vi "deserialize (Frames-AIM).vi"(11 "data in":string[][](array[string])) -> (3 "frames":map{string, map{string, T1}}[](array[numeric]))   [LabVIEW 2020]
uses:
  _controls/1553_minorFrames.ctl
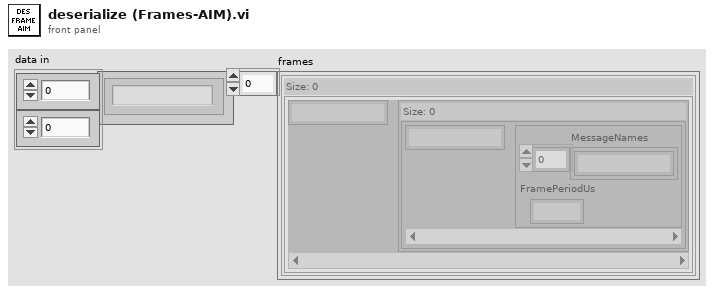
[diagram p1: front panel]
types:
  T1 = typedef "1553_minorFrames.ctl" = cluster{"MessageNames":string[], "FramePeriodUs":i32}
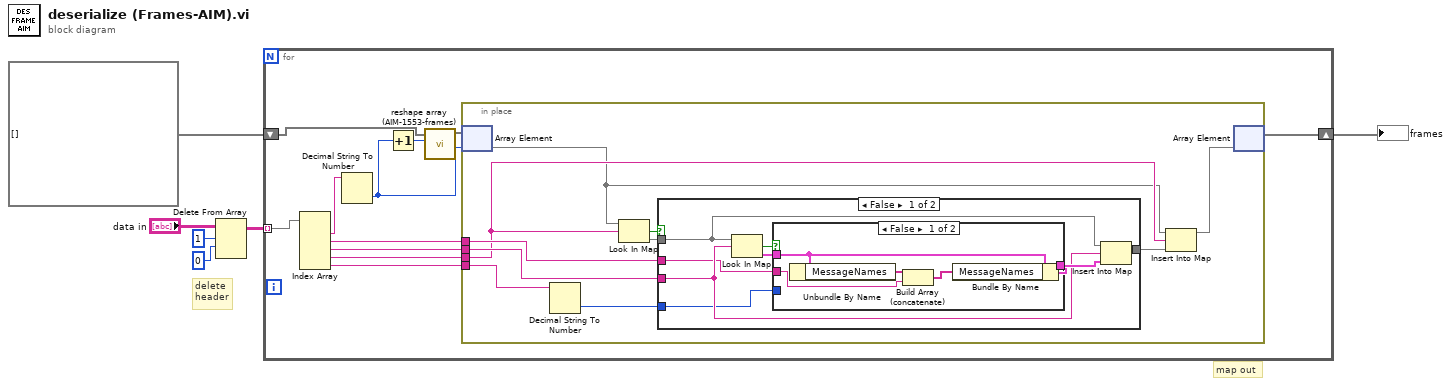
[diagram p0: block diagram]
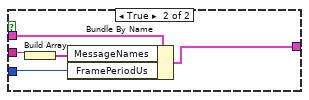
[diagram p2: hidden frame]
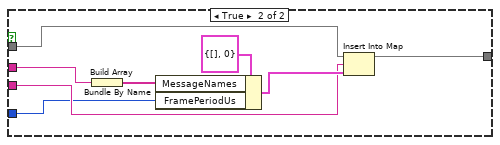
[diagram p3: hidden frame]
diagram:
  # "delete\nheader"
  # "map out"
  n1 = Delete From Array(array="data in", length=1, index (row)=0) -> (array with subset deleted=w3:string[][])  [unwired: 1 in, 1 out]
  n2 = for {
    tunnel: w3 -> [w17] mode=indexing
    shift-right: [w12] -> w1
    shift-left: map{string, map{string, T1}}[] [] ("map") -> [w11]
    n3 = Index Array(array=w17) -> (element #1=w10:string, element #2=w15:string, element #3=w14:string, element #4=w13:string, element #5=w16:string)  [unwired: 5 in]
    n4 = Decimal String To Number(string=w10) -> (number=w8:i32)  [unwired: 2 in, 1 out]
    n5 = Increment(x=w8) -> (x+1=w7:i32)
    n6 = call "reshape array (AIM-1553-frames).vi"("index requested"=w7, "map array in"=w11) -> ("map array out"=w9:map{string, map{string, T1}}[])  [unwired: 9 in]
    n7 = in-place {
      in-place-border: w16 -> [w27]
      in-place-border: w15 -> [w25]
      in-place-border: w14 -> [w24]
      in-place-border: w13 -> [w21]
      n8 = in-place-array #1(w9, w8) -> (w19:map{string, map{string, T1}})
      n9 = Decimal String To Number(string=w27) -> (number=w23:i32)  [unwired: 2 in, 1 out]
      n10 = Look In Map(map=w19, key=w21) -> (key not found?=w26:bool, value=w22:map{string, T1})  [unwired: 1 in]
      n11 = case shown="False" w26 {
        tunnel: w25 -> [w29 w49]
        tunnel: w24 -> [w31 w47]
        tunnel: w23 -> [w28 w46]
        tunnel: w22 -> [w33 w53]
        tunnel: [w30 w52] -> w20
        frame False {
          n12 = Look In Map(map=w33, key=w31) -> (key not found?=w35:bool, value=w34:T1)  [unwired: 1 in]
          n13 = case shown="False" w35 {
            tunnel: w34 -> [w40 w45]
            tunnel: w28 -> [_ w44]
            tunnel: w29 -> [w36 w43]
            tunnel: [w39 w41] -> w32
            frame False {
              n14 = Unbundle By Name(w40) -> ("MessageNames"=w38:string[])
              n15 = Build Array (concatenate)(w38, w36) -> (w37:string[])
              n16 = Bundle By Name(cluster=w40, "MessageNames"=w37) -> (w39:T1)
            }
            frame True {
              n17 = Build Array(w43) -> (w42:string[])
              n18 = Bundle By Name(cluster=w45, "MessageNames"=w42, "FramePeriodUs"=w44) -> (w41:T1)
            }
          }
          n19 = Insert Into Map(map in=w33, key=w31, value=w32) -> (map out=w30:map{string, T1})  [unwired: 2 out]
        }
        frame True {
          n20 = Build Array(w49) -> (w48:string[])
          n21 = Bundle By Name(cluster=T1 {"MessageNames"=[], "FramePeriodUs"=0} ("value"), "MessageNames"=w48, "FramePeriodUs"=w46) -> (w50:T1)
          n22 = Insert Into Map(map in=w53, key=w47, value=w50) -> (map out=w52:map{string, T1})  [unwired: 2 out]
        }
      }
      n23 = Insert Into Map(map in=w19, key=w21, value=w20) -> (map out=w18:map{string, map{string, T1}})  [unwired: 2 out]
      n24 = in-place-array #1(w18) -> (w12:map{string, map{string, T1}}[])  [unwired: 1 out]
    }
  }
  "frames" <- w1
